vi "Disconnect.vi"(8 "error in (no error)":errorcluster, 11 "ImageHandler in":refnum<class "ImageHandler.lvclass">) -> (0 "error out":errorcluster, 3 "ImageHandler out":refnum<class "ImageHandler.lvclass">)   [LabVIEW 2022 SP3, in "ImageHandler.lvlib" / "ImageHandler.lvclass"]
uses:
  ImageHandler.lvclass
  ImageHandler.lvclass/ImageHandler.ctl
  BonTechDetector/BonTechDetector.lvlib
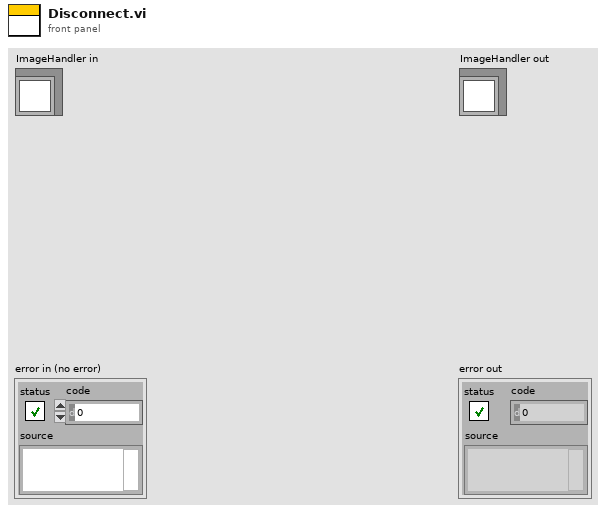
[diagram p1: front panel]
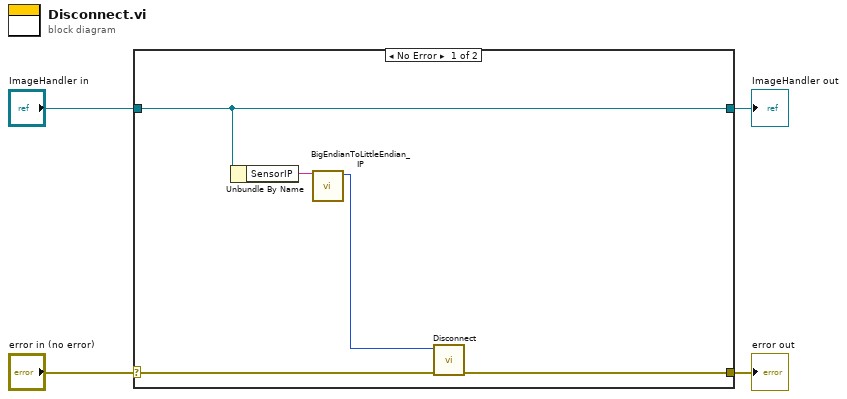
[diagram p0: block diagram]
diagram:
  n1 = case shown="No Error" "error in (no error)" {
    selector: "error in (no error)" -> [w6 w11]
    tunnel: [w5 w11] -> w3
    tunnel: [w9 w10] -> w1
    tunnel: "ImageHandler in" -> [w9 w10]
    frame No Error {
      n2 = Unbundle By Name(w9) -> ("SensorIP"=w8:string)
      n3 = call "BigEndianToLittleEndian_IP.vi"("IP String"=w8) -> ("IP Network Order"=w7:u32)  [unwired: 10 in]
      n4 = call "Disconnect.vi"("error in (no error)"=w6, "nSensorIP"=w7) -> ("error out"=w5:errorcluster)  [unwired: 8 in, 1 out]
    }
    frame Error {
    }
  }
  "error out" <- w3
  "ImageHandler out" <- w1
